vi "SanityChecker-Pressures.vi"(7 "Minimum dP":dbl=0.2, 11 "ZeroedPressures":dbl[][](array[numeric])) -> (1 "GoodPressures":T2, 3 "Sanity":T1={"PressureErrors"=[], "Plug in titles"=["Good", "AllNegative", "dPTooSmall", "P1smallest", "FailedToReduce", "ExceedMaxCone", "U.LT.0"]})   [LabVIEW 2016]
uses:
  GoodArray.ctl
  SanityCluster.ctl
panel:
  # "#Warning !!Not relevant for Omniprobe!!"
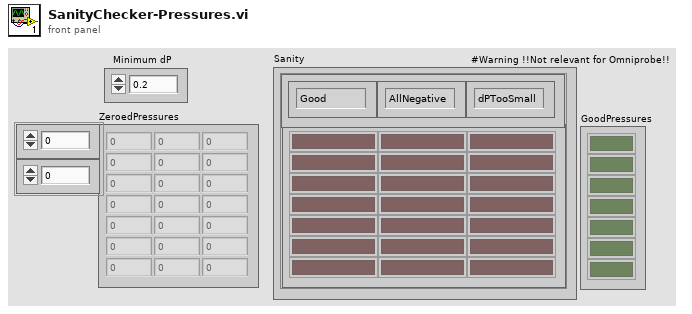
[diagram p1: front panel]
types:
  T1 = typedef "SanityCluster.ctl" = cluster{"PressureErrors":bool[][], "Plug in titles":string[]}
  T2 = typedef "GoodArray.ctl" = bool[]
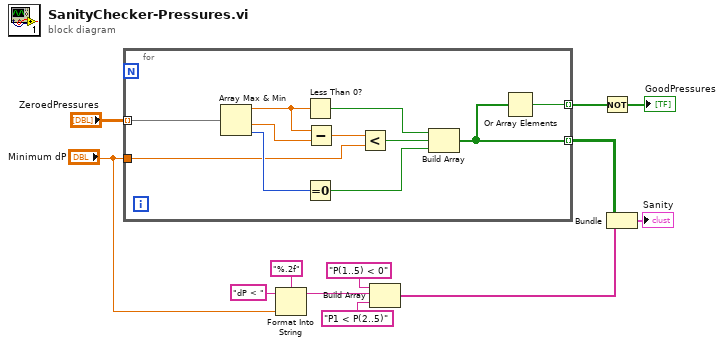
[diagram p0: block diagram]
diagram:
  n1 = for {
    tunnel: "ZeroedPressures" -> [w17] mode=indexing
    tunnel: [w15] -> w3 mode=indexing
    tunnel: [w14] -> w11 mode=indexing
    tunnel: "Minimum dP" -> [w13]
    n2 = Array Max & Min(array=w17) -> (max value=w18:dbl, min value=w19:dbl, min index (indices)=w22:i32)  [unwired: 1 out]
    n3 = Less Than 0?(x=w18) -> (x < 0?=w23:bool)
    n4 = Equal To 0?(x=w22) -> (x = 0?=w16:bool)
    n5 = Subtract(x=w18, y=w19) -> (x-y=w20:dbl)
    n6 = Less?(x=w20, y=w13) -> (x < y?=w21:bool)
    n7 = Build Array(w23, w21, w16) -> (w15:bool[])
    n8 = Or Array Elements(Boolean array=w15) -> (logical OR=w14:bool)
  }
  n9 = Format Into String(format string="%.2f", initial string="dP < ", "Minimum dP") -> (resulting string=w5:string)  [unwired: 1 in, 1 out]
  n10 = Build Array("P(1..5) < 0", w5, "P1 < P(2..5)") -> (w2:string[])
  n11 = Not(x=w11) -> (.not. x?=→"GoodPressures":bool[])
  n12 = Bundle(w3, w2) -> (→"Sanity":cluster{bool[][], string[]})  [unwired: 1 in]
